vi "Get Multi t0 on Variant.vi"(8 "error in (no error)":errorcluster, 11 "Variant in":variant) -> (0 "error out":errorcluster, 2 "t0s":timestamp[](array[timestamp]), 3 "Variant out":variant)   [LabVIEW 2020, in "Internal Comm Classes.lvlib" / "WPL Comm.lvclass"]
uses:
  WPL Comm.lvclass
  <vilib>/Utility/error.llb/Error Cluster From Error Code.vi
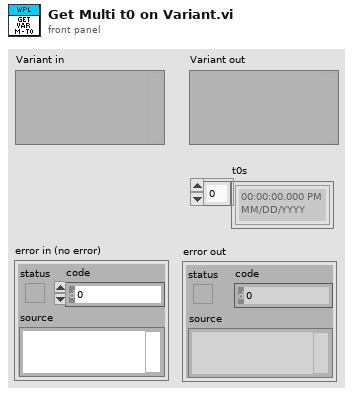
[diagram p1: front panel]
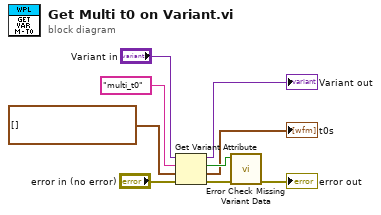
[diagram p0: block diagram]
diagram:
  n1 = Get Variant Attribute(Variant="Variant in", name="multi_t0", default value (empty Variant)=timestamp[] [], error in="error in (no error)") -> (duplicate Variant=→"Variant out":variant, found=w5:bool, value=→"t0s":timestamp[], error out=w4:errorcluster)
  n2 = call "Error Check Missing Variant Data.vi"("error in (no error)"=w4, "Found?"=w5) -> ("error out"=→"error out":errorcluster)  [unwired: 9 in]
